vi "窗口是否在最前.vi"(8 "错误输入（无错误）":errorcluster, 11 "引用":refnum<vi>) -> (0 "错误输出":errorcluster, 2 "在最前？":bool, 3 "引用输出":refnum<vi>)   [LabVIEW 8.6, in "窗口操作.lvlib"]
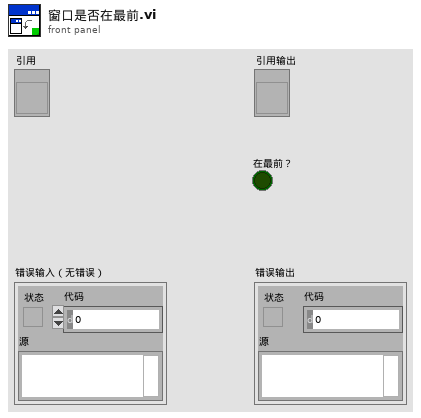
[diagram p1: front panel]
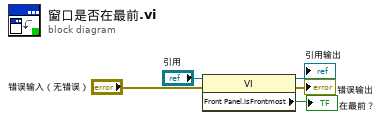
[diagram p0: block diagram]
diagram:
  n1 = property class="VI"(reference="引用", error in="错误输入（无错误）") -> (reference out=→"引用输出":refnum<vi>, error out=→"错误输出":errorcluster, "Front Panel.IsFrontmost"=→"在最前？":bool)
